vi "WILT Send Start Stop CMD.vi"(0 "Dryer Step 4 In":T5 {"Night Cycle Count" format="%04d"; "Day Cycle Count" format="%04d"}, 2 "Step 3 Input":T3, 3 "Final Start Presses":i32=2, 5 "Error In":errorcluster, 7 "Current Threshold":dbl, 8 "Station Number in":u32, 9 "Agilent Valve and Switch Locations":T2[](array[typedef])=[{"Channel"="301", "Station"="1", "Label"="Water Valve", "Agilent Station"="2", "Data"=0.0}, {"Channel"="302", "Station"="2", "Label"="Water Valve", "Agilent Station"="2", "Data"=0.0}, {"Channel"="303", "Station"="3", "Label"="Water Valve", "Agilent Station"="2", "Data"=0.0}, {"Channel"="304", "Station"="4", "Label"="Water Valve", "Agilent Station"="2", "Data"=0.0}, {"Channel"="305", "Station"="5", "Label"="Water Valve", "Agilent Station"="2", "Data"=0.0}, {"Channel"="306", "Station"="6", "Label"="Water Valve", "Agilent Station"="2", "Data"=0.0}, {"Channel"="307", "Station"="7", "Label"="Water Valve", "Agilent Station"="2", "Data"=0.0}, {"Channel"="308", "Station"="8", "Label"="Water Valve", "Agilent Station"="2", "Data"=0.0}, {"Channel"="309", "Station"="9", "Label"="Water Valve", "Agilent Station"="2", "Data"=0.0}, {"Channel"="310", "Station"="10", "Label"="Water Valve", "Agilent Station"="2", "Data"=0.0}, {"Channel"="311", "Station"="11", "Label"="Water Valve", "Agilent Station"="2", "Data"=0.0}, {"Channel"="312", "Station"="12", "Label"="Water Valve", "Agilent Station"="2", "Data"=0.0}, {"Channel"="313", "Station"="13", "Label"="Water Valve", "Agilent Station"="2", "Data"=0.0}, {"Channel"="314", "Station"="14", "Label"="Water Valve", "Agilent Station"="2", "Data"=0.0}, {"Channel"="315", "Station"="15", "Label"="Water Valve", "Agilent Station"="2", "Data"=0.0}, {"Channel"="316", "Station"="16", "Label"="Water Valve", "Agilent Station"="2", "Data"=0.0}, {"Channel"="317", "Station"="17", "Label"="Water Valve", "Agilent Station"="2", "Data"=0.0}, {"Channel"="318", "Station"="18", "Label"="Water Valve", "Agilent Station"="2", "Data"=0.0}, {"Channel"="319", "Station"="19", "Label"="Water Valve", "Agilent Station"="2", "Data"=0.0}, {"Channel"="320", "Station"="20", "Label"="Water Valve", "Agilent Station"="2", "Data"=0.0}, {"Channel"="101", "Station"="21", "Label"="Water Valve", "Agilent Station"="3", "Data"=0.0}, {"Channel"="102", "Station"="22", "Label"="Water Valve", "Agilent Station"="3", "Data"=0.0}, {"Channel"="103", "Station"="23", "Label"="Water Valve", "Agilent Station"="3", "Data"=0.0}, {"Channel"="104", "Station"="24", "Label"="Water Valve", "Agilent Station"="3", "Data"=0.0}, {"Channel"="105", "Station"="25", "Label"="Water Valve", "Agilent Station"="3", "Data"=0.0}, {"Channel"="106", "Station"="26", "Label"="Water Valve", "Agilent Station"="3", "Data"=0.0}, {"Channel"="107", "Station"="27", "Label"="Water Valve", "Agilent Station"="3", "Data"=0.0}, {"Channel"="108", "Station"="28", "Label"="Water Valve", "Agilent Station"="3", "Data"=0.0}, {"Channel"="109", "Station"="29", "Label"="Water Valve", "Agilent Station"="3", "Data"=0.0}, {"Channel"="110", "Station"="30", "Label"="Water Valve", "Agilent Station"="3", "Data"=0.0}, {"Channel"="111", "Station"="31", "Label"="Water Valve", "Agilent Station"="3", "Data"=0.0}, {"Channel"="112", "Station"="32", "Label"="Water Valve", "Agilent Station"="3", "Data"=0.0}, {"Channel"="101", "Station"="33", "Label"="Water Valve", "Agilent Station"="5", "Data"=0.0}, {"Channel"="102", "Station"="34", "Label"="Water Valve", "Agilent Station"="5", "Data"=0.0}, {"Channel"="103", "Station"="35", "Label"="Water Valve", "Agilent Station"="5", "Data"=0.0}, {"Channel"="104", "Station"="36", "Label"="Water Valve", "Agilent Station"="5", "Data"=0.0}, {"Channel"="105", "Station"="37", "Label"="Water Valve", "Agilent Station"="5", "Data"=0.0}, {"Channel"="106", "Station"="38", "Label"="Water Valve", "Agilent Station"="5", "Data"=0.0}, {"Channel"="107", "Station"="39", "Label"="Water Valve", "Agilent Station"="5", "Data"=0.0}, {"Channel"="108", "Station"="40", "Label"="Water Valve", "Agilent Station"="5", "Data"=0.0}, {"Channel"="109", "Station"="41", "Label"="Water Valve", "Agilent Station"="5", "Data"=0.0}, {"Channel"="110", "Station"="42", "Label"="Water Valve", "Agilent Station"="5", "Data"=0.0}, {"Channel"="111", "Station"="43", "Label"="Water Valve", "Agilent Station"="5", "Data"=0.0}, {"Channel"="112", "Station"="44", "Label"="Water Valve", "Agilent Station"="5", "Data"=0.0}, {"Channel"="113", "Station"="45", "Label"="Water Valve", "Agilent Station"="5", "Data"=0.0}, {"Channel"="114", "Station"="46", "Label"="Water Valve", "Agilent Station"="5", "Data"=0.0}, {"Channel"="115", "Station"="47", "Label"="Water Valve", "Agilent Station"="5", "Data"=0.0}, {"Channel"="116", "Station"="48", "Label"="Water Valve", "Agilent Station"="5", "Data"=0.0}, {"Channel"="117", "Station"="49", "Label"="Water Valve", "Agilent Station"="5", "Data"=0.0}, {"Channel"="118", "Station"="50", "Label"="Water Valve", "Agilent Station"="5", "Data"=0.0}, {"Channel"="119", "Station"="51", "Label"="Water Valve", "Agilent Station"="5", "Data"=0.0}, {"Channel"="120", "Station"="52", "Label"="Water Valve", "Agilent Station"="5", "Data"=0.0}, {"Channel"="201", "Station"="53", "Label"="Water Valve", "Agilent Station"="5", "Data"=0.0}, {"Channel"="202", "Station"="54", "Label"="Water Valve", "Agilent Station"="5", "Data"=0.0}, {"Channel"="203", "Station"="55", "Label"="Water Valve", "Agilent Station"="5", "Data"=0.0}, {"Channel"="204", "Station"="56", "Label"="Water Valve", "Agilent Station"="5", "Data"=0.0}, {"Channel"="301", "Station"="21", "Label"="Start Button", "Agilent Station"="5", "Data"=0.0}, {"Channel"="302", "Station"="22", "Label"="Start Button", "Agilent Station"="5", "Data"=0.0}, {"Channel"="303", "Station"="23", "Label"="Start Button", "Agilent Station"="5", "Data"=0.0}, {"Channel"="304", "Station"="24", "Label"="Start Button", "Agilent Station"="5", "Data"=0.0}, {"Channel"="305", "Station"="25", "Label"="Start Button", "Agilent Station"="5", "Data"=0.0}, {"Channel"="306", "Station"="26", "Label"="Start Button", "Agilent Station"="5", "Data"=0.0}, {"Channel"="307", "Station"="27", "Label"="Start Button", "Agilent Station"="5", "Data"=0.0}, {"Channel"="308", "Station"="28", "Label"="Start Button", "Agilent Station"="5", "Data"=0.0}, {"Channel"="309", "Station"="29", "Label"="Start Button", "Agilent Station"="5", "Data"=0.0}, {"Channel"="310", "Station"="30", "Label"="Start Button", "Agilent Station"="5", "Data"=0.0}, {"Channel"="311", "Station"="31", "Label"="Start Button", "Agilent Station"="5", "Data"=0.0}, {"Channel"="312", "Station"="32", "Label"="Start Button", "Agilent Station"="5", "Data"=0.0}, {"Channel"="101", "Station"="33", "Label"="Start Button", "Agilent Station"="7", "Data"=0.0}, {"Channel"="102", "Station"="34", "Label"="Start Button", "Agilent Station"="7", "Data"=0.0}, {"Channel"="103", "Station"="35", "Label"="Start Button", "Agilent Station"="7", "Data"=0.0}, {"Channel"="104", "Station"="36", "Label"="Start Button", "Agilent Station"="7", "Data"=0.0}, {"Channel"="105", "Station"="37", "Label"="Start Button", "Agilent Station"="7", "Data"=0.0}, {"Channel"="106", "Station"="38", "Label"="Start Button", "Agilent Station"="7", "Data"=0.0}, {"Channel"="107", "Station"="39", "Label"="Start Button", "Agilent Station"="7", "Data"=0.0}, {"Channel"="108", "Station"="40", "Label"="Start Button", "Agilent Station"="7", "Data"=0.0}, {"Channel"="109", "Station"="41", "Label"="Start Button", "Agilent Station"="7", "Data"=0.0}, {"Channel"="110", "Station"="42", "Label"="Start Button", "Agilent Station"="7", "Data"=0.0}, {"Channel"="111", "Station"="43", "Label"="Start Button", "Agilent Station"="7", "Data"=0.0}, {"Channel"="112", "Station"="44", "Label"="Start Button", "Agilent Station"="7", "Data"=0.0}, {"Channel"="113", "Station"="45", "Label"="Start Button", "Agilent Station"="7", "Data"=0.0}, {"Channel"="114", "Station"="46", "Label"="Start Button", "Agilent Station"="7", "Data"=0.0}, {"Channel"="115", "Station"="47", "Label"="Start Button", "Agilent Station"="7", "Data"=0.0}, {"Channel"="116", "Station"="48", "Label"="Start Button", "Agilent Station"="7", "Data"=0.0}, {"Channel"="117", "Station"="49", "Label"="Start Button", "Agilent Station"="7", "Data"=0.0}, {"Channel"="118", "Station"="50", "Label"="Start Button", "Agilent Station"="7", "Data"=0.0}, {"Channel"="119", "Station"="51", "Label"="Start Button", "Agilent Station"="7", "Data"=0.0}, {"Channel"="120", "Station"="52", "Label"="Start Button", "Agilent Station"="7", "Data"=0.0}, {"Channel"="201", "Station"="53", "Label"="Start Button", "Agilent Station"="7", "Data"=0.0}, {"Channel"="202", "Station"="54", "Label"="Start Button", "Agilent Station"="7", "Data"=0.0}, {"Channel"="203", "Station"="55", "Label"="Start Button", "Agilent Station"="7", "Data"=0.0}, {"Channel"="204", "Station"="56", "Label"="Start Button", "Agilent Station"="7", "Data"=0.0}], 13 "Semaphore":T1[](array[typedef])) -> (14 "Dryer Step 4 Output":T5 {"Night Cycle Count" format="%04d"; "Day Cycle Count" format="%04d"}, 16 "Step 3 Output":T3, 19 "Error Out":errorcluster)   [LabVIEW 2016]
uses:
  Type Definitions/WILT Station Test State Cluster.ctl
  Type Definitions/WILT Dryer Test State.ctl
  Type Definitions/WILT Dryer.ctl
  Type Definitions/WILT Dryer Details.ctl
  Type Definitions/WILT Agilent Channel Definition.ctl
  Type Definitions/WILT DAQ Data.ctl
  Globals/WILT Globals Main Program.vi
panel:
  # "Day"
  # "Night"
  # "Day"
  # "Night"
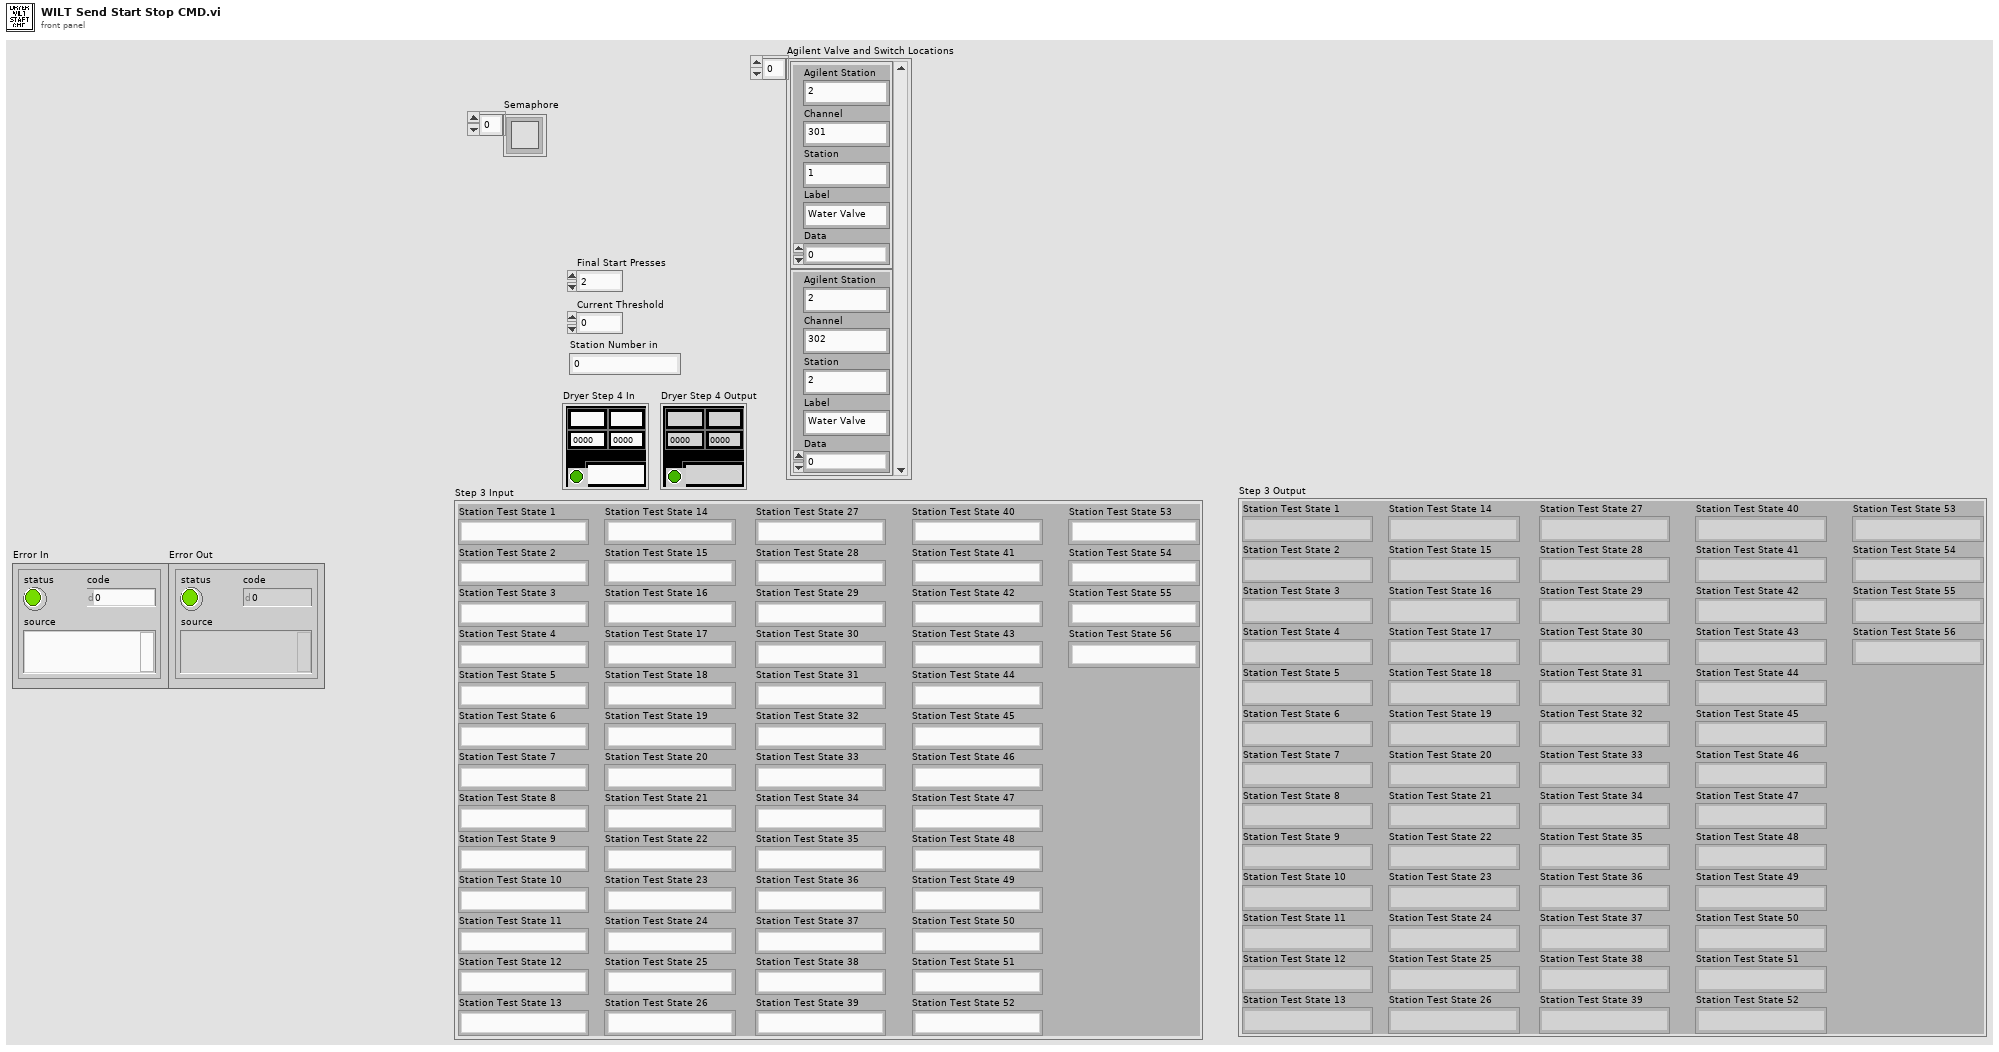
[diagram p1: front panel]
types:
  T1 = typedef "Semaphore RefNum" = refnum<k1>
  T2 = typedef "WILT Agilent Channel Definition.ctl" = cluster{"Channel":string, "Station":string, "Label":string, "Agilent Station":string, "Data":dbl}
  T3 = typedef "WILT Station Test State Cluster.ctl" = cluster{"Station Test State 1":T4, "Station Test State 2":T4, "Station Test State 3":T4, "Station Test State 4":T4, "Station Test State 5":T4, "Station Test State 6":T4, "Station Test State 7":T4, "Station Test State 8":T4, "Station Test State 9":T4, "Station Test State 10":T4, "Station Test State 11":T4, "Station Test State 12":T4, "Station Test State 13":T4, "Station Test State 14":T4, "Station Test State 15":T4, "Station Test State 16":T4, "Station Test State 17":T4, "Station Test State 18":T4, "Station Test State 19":T4, "Station Test State 20":T4, "Station Test State 21":T4, "Station Test State 22":T4, "Station Test State 23":T4, "Station Test State 24":T4, "Station Test State 25":T4, "Station Test State 26":T4, "Station Test State 27":T4, "Station Test State 28":T4, "Station Test State 29":T4, "Station Test State 30":T4, "Station Test State 31":T4, "Station Test State 32":T4, "Station Test State 33":T4, "Station Test State 34":T4, "Station Test State 35":T4, "Station Test State 36":T4, "Station Test State 37":T4, "Station Test State 38":T4, "Station Test State 39":T4, "Station Test State 40":T4, "Station Test State 41":T4, "Station Test State 42":T4, "Station Test State 43":T4, "Station Test State 44":T4, "Station Test State 45":T4, "Station Test State 46":T4, "Station Test State 47":T4, "Station Test State 48":T4, "Station Test State 49":T4, "Station Test State 50":T4, "Station Test State 51":T4, "Station Test State 52":T4, "Station Test State 53":T4, "Station Test State 54":T4, "Station Test State 55":T4, "Station Test State 56":T4}
  T4 = typedef "WILT Dryer Test State.ctl" = enum16{"No Serial Number", "Waiting for Dryer To Start", "Drying Clothes", "Water Injection 1 (On)", "Water Injection 1 Timer", "Water Injection 1 (Off)", "Pause Dryer", "Sending Start Stop CMD", "Pause Dryer 2", "Sending Start Stop CMD 2", "Drying Clothes 2", "Water Injection 2 (On)", "Water Injection 2 Timer", "Water Injection 2 (Off)", "Drying Clothes 3", "Cooling Down", "Sending Start Stop CMD 3", "Increment Cycle"}
  T5 = typedef "WILT Dryer.ctl" = cluster{"Lab ID":string, "Day Cycle Count":i32, "Station Label":string, "Dryer Details":T6, "Status Color":u32, "Invisible Button":bool, "Night Cycle Count":i32, "Station Index":i32, "Cycle Index":string, "Audit Alert":bool, "Agilent Channel Definition":T2, "DAQ Data":T7}
  T6 = typedef "WILT Dryer Details.ctl" = cluster{"Station":string, "Lab ID":string, "TR Number":string}
  T7 = typedef "WILT DAQ Data.ctl" = cluster{"L1 Current":dbl, "L2 Current":dbl, "Temperature  Deg F (TC)":dbl, "Volts":dbl, "Volts (208)":dbl, "SW (208)":dbl}
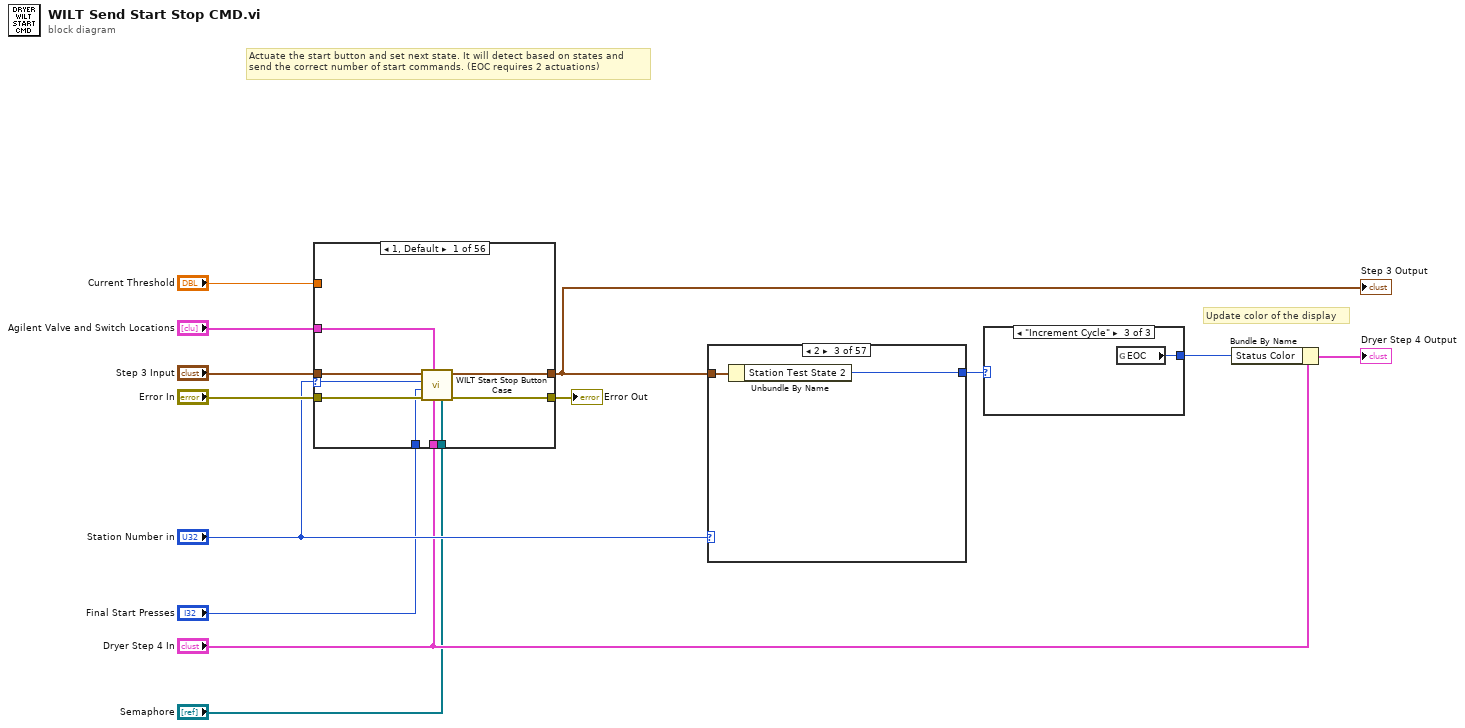
[diagram p0: block diagram]
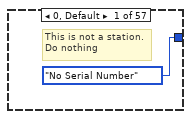
[diagram p2: hidden frame]
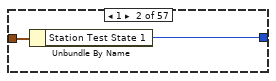
[diagram p3: hidden frame]
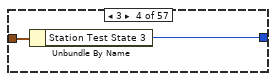
[diagram p4: hidden frame]
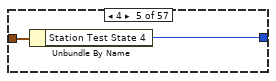
[diagram p5: hidden frame]
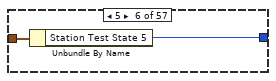
[diagram p6: hidden frame]
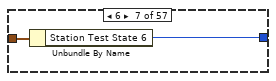
[diagram p7: hidden frame]
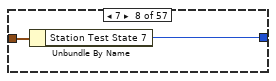
[diagram p8: hidden frame]
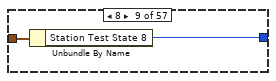
[diagram p9: hidden frame]
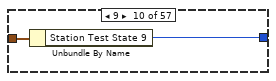
[diagram p10: hidden frame]
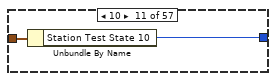
[diagram p11: hidden frame]
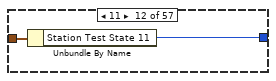
[diagram p12: hidden frame]
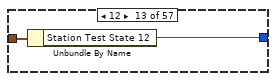
[diagram p13: hidden frame]
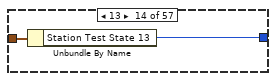
[diagram p14: hidden frame]
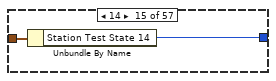
[diagram p15: hidden frame]
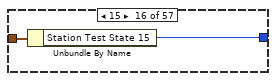
[diagram p16: hidden frame]
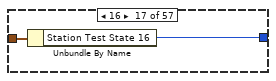
[diagram p17: hidden frame]
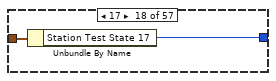
[diagram p18: hidden frame]
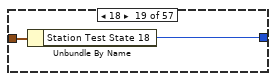
[diagram p19: hidden frame]
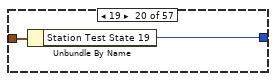
[diagram p20: hidden frame]
diagram:
  # "Update color of the display"
  # "Actuate the start button and set next state. It will detect based on states and \nsend the correct number of start commands. (EOC requires 2 actuations)"
  n1 = case shown="1, Default" "Station Number in" {
    selector: "Station Number in" -> [w20 w30 w38 w49 w58 w64 w72 w81 w90 w102 w109 w117 w128 w135 w144 w153 w162 w173 w180 w189 w198 w207 w216 w225 w238 w245 w254 w261 w273 w282 w290 w297 w309 w315 w324 w336 w342 w351 w360 w369 w380 w387 w399 w407 w416 w423 w432 w444 w450 w459 w468 w480 w486 w495 w504 w517]
    tunnel: "Step 3 Input" -> [w22 w31 w40 w48 w57 w65 w76 w85 w94 w103 w112 w121 w127 w139 w146 w157 w166 w175 w184 w193 w202 w211 w220 w229 w235 w247 w256 w265 w274 w283 w292 w301 w310 w319 w328 w337 w346 w355 w364 w371 w382 w391 w400 w409 w418 w427 w436 w445 w454 w463 w472 w481 w490 w499 w508 w516]
    tunnel: [w21 w27 w39 w47 w54 w63 w75 w84 w93 w99 w111 w120 w126 w136 w145 w156 w164 w172 w183 w192 w201 w210 w219 w228 w234 w244 w255 w264 w270 w279 w289 w300 w306 w318 w325 w333 w345 w354 w363 w370 w381 w390 w396 w408 w417 w426 w435 w441 w453 w462 w471 w477 w489 w498 w507 w515] -> w9
    tunnel: "Error In" -> [w19 w29 w37 w46 w56 w67 w73 w82 w91 w101 w110 w118 w130 w138 w148 w154 w165 w174 w181 w190 w199 w208 w217 w226 w237 w246 w253 w262 w272 w281 w291 w298 w308 w316 w327 w335 w343 w352 w361 w373 w379 w388 w398 w406 w415 w424 w433 w443 w451 w461 w469 w479 w487 w496 w505 w514]
    tunnel: [w18 w28 w36 w45 w55 w66 w74 w83 w92 w100 w108 w119 w129 w137 w147 w155 w163 w171 w182 w191 w200 w209 w218 w227 w236 w243 w252 w263 w271 w280 w288 w299 w307 w317 w326 w334 w344 w353 w362 w372 w378 w389 w397 w405 w414 w425 w434 w442 w452 w460 w470 w478 w488 w497 w506 w513] -> w10
    tunnel: "Agilent Valve and Switch Locations" -> [w17 w26 w35 w44 w53 w62 w71 w80 w89 w98 w107 w116 w125 w134 w143 w152 w161 w170 w179 w188 w197 w206 w215 w224 w233 w242 w251 w260 w269 w278 w287 w296 w305 w314 w323 w332 w341 w350 w359 w368 w377 w386 w395 w404 w413 w422 w431 w440 w449 w458 w467 w476 w485 w494 w503 w512]
    tunnel: "Current Threshold" -> [_ _ _ _ _ _ _ _ _ _ _ _ _ _ _ _ _ _ _ _ _ _ _ _ _ _ _ _ _ _ _ _ _ _ _ _ _ _ _ _ _ _ _ _ _ _ _ _ _ _ _ _ _ _ _ _]
    tunnel: "Dryer Step 4 In" -> [w16 w25 w34 w43 w52 w61 w70 w79 w88 w97 w106 w115 w124 w133 w142 w151 w160 w169 w178 w187 w196 w205 w214 w223 w232 w241 w250 w259 w268 w277 w286 w295 w304 w313 w322 w331 w340 w349 w358 w367 w376 w385 w394 w403 w412 w421 w430 w439 w448 w457 w466 w475 w484 w493 w502 w511]
    tunnel: "Semaphore" -> [w15 w24 w33 w42 w51 w60 w69 w78 w87 w96 w105 w114 w123 w132 w141 w150 w159 w168 w177 w186 w195 w204 w213 w222 w231 w240 w249 w258 w267 w276 w285 w294 w303 w312 w321 w330 w339 w348 w357 w366 w375 w384 w393 w402 w411 w420 w429 w438 w447 w456 w465 w474 w483 w492 w501 w510]
    tunnel: "Final Start Presses" -> [w14 w23 w32 w41 w50 w59 w68 w77 w86 w95 w104 w113 w122 w131 w140 w149 w158 w167 w176 w185 w194 w203 w212 w221 w230 w239 w248 w257 w266 w275 w284 w293 w302 w311 w320 w329 w338 w347 w356 w365 w374 w383 w392 w401 w410 w419 w428 w437 w446 w455 w464 w473 w482 w491 w500 w509]
    frame 1, Default {
      n2 = call "WILT Start Stop Button Case.vi"("Semaphore"=w15, "Dryer Step 4 In"=w16, "Agilent Valve and Switch Locations"=w17, "Error In"=w19, "Final Start Presses"=w14, "Station Number"=w20, "Step 3 Input in"=w22) -> ("Error Out"=w18:errorcluster, "Step 3 Input out"=w21:T3)  [unwired: 3 in]
    }
    frame 2 {
      n3 = call "WILT Start Stop Button Case.vi"("Semaphore"=w24, "Dryer Step 4 In"=w25, "Agilent Valve and Switch Locations"=w26, "Error In"=w29, "Final Start Presses"=w23, "Station Number"=w30, "Step 3 Input in"=w31) -> ("Error Out"=w28:errorcluster, "Step 3 Input out"=w27:T3)  [unwired: 3 in]
    }
    frame 3 {
      n4 = call "WILT Start Stop Button Case.vi"("Semaphore"=w33, "Dryer Step 4 In"=w34, "Agilent Valve and Switch Locations"=w35, "Error In"=w37, "Final Start Presses"=w32, "Station Number"=w38, "Step 3 Input in"=w40) -> ("Error Out"=w36:errorcluster, "Step 3 Input out"=w39:T3)  [unwired: 3 in]
    }
    frame 4 {
      n5 = call "WILT Start Stop Button Case.vi"("Semaphore"=w42, "Dryer Step 4 In"=w43, "Agilent Valve and Switch Locations"=w44, "Error In"=w46, "Final Start Presses"=w41, "Station Number"=w49, "Step 3 Input in"=w48) -> ("Error Out"=w45:errorcluster, "Step 3 Input out"=w47:T3)  [unwired: 3 in]
    }
    frame 5 {
      n6 = call "WILT Start Stop Button Case.vi"("Semaphore"=w51, "Dryer Step 4 In"=w52, "Agilent Valve and Switch Locations"=w53, "Error In"=w56, "Final Start Presses"=w50, "Station Number"=w58, "Step 3 Input in"=w57) -> ("Error Out"=w55:errorcluster, "Step 3 Input out"=w54:T3)  [unwired: 3 in]
    }
    frame 6 {
      n7 = call "WILT Start Stop Button Case.vi"("Semaphore"=w60, "Dryer Step 4 In"=w61, "Agilent Valve and Switch Locations"=w62, "Error In"=w67, "Final Start Presses"=w59, "Station Number"=w64, "Step 3 Input in"=w65) -> ("Error Out"=w66:errorcluster, "Step 3 Input out"=w63:T3)  [unwired: 3 in]
    }
    frame 7 {
      n8 = call "WILT Start Stop Button Case.vi"("Semaphore"=w69, "Dryer Step 4 In"=w70, "Agilent Valve and Switch Locations"=w71, "Error In"=w73, "Final Start Presses"=w68, "Station Number"=w72, "Step 3 Input in"=w76) -> ("Error Out"=w74:errorcluster, "Step 3 Input out"=w75:T3)  [unwired: 3 in]
    }
    frame 8 {
      n9 = call "WILT Start Stop Button Case.vi"("Semaphore"=w78, "Dryer Step 4 In"=w79, "Agilent Valve and Switch Locations"=w80, "Error In"=w82, "Final Start Presses"=w77, "Station Number"=w81, "Step 3 Input in"=w85) -> ("Error Out"=w83:errorcluster, "Step 3 Input out"=w84:T3)  [unwired: 3 in]
    }
    frame 9 {
      n10 = call "WILT Start Stop Button Case.vi"("Semaphore"=w87, "Dryer Step 4 In"=w88, "Agilent Valve and Switch Locations"=w89, "Error In"=w91, "Final Start Presses"=w86, "Station Number"=w90, "Step 3 Input in"=w94) -> ("Error Out"=w92:errorcluster, "Step 3 Input out"=w93:T3)  [unwired: 3 in]
    }
    frame 10 {
      n11 = call "WILT Start Stop Button Case.vi"("Semaphore"=w96, "Dryer Step 4 In"=w97, "Agilent Valve and Switch Locations"=w98, "Error In"=w101, "Final Start Presses"=w95, "Station Number"=w102, "Step 3 Input in"=w103) -> ("Error Out"=w100:errorcluster, "Step 3 Input out"=w99:T3)  [unwired: 3 in]
    }
    frame 11 {
      n12 = call "WILT Start Stop Button Case.vi"("Semaphore"=w105, "Dryer Step 4 In"=w106, "Agilent Valve and Switch Locations"=w107, "Error In"=w110, "Final Start Presses"=w104, "Station Number"=w109, "Step 3 Input in"=w112) -> ("Error Out"=w108:errorcluster, "Step 3 Input out"=w111:T3)  [unwired: 3 in]
    }
    frame 12 {
      n13 = call "WILT Start Stop Button Case.vi"("Semaphore"=w114, "Dryer Step 4 In"=w115, "Agilent Valve and Switch Locations"=w116, "Error In"=w118, "Final Start Presses"=w113, "Station Number"=w117, "Step 3 Input in"=w121) -> ("Error Out"=w119:errorcluster, "Step 3 Input out"=w120:T3)  [unwired: 3 in]
    }
    frame 13 {
      n14 = call "WILT Start Stop Button Case.vi"("Semaphore"=w123, "Dryer Step 4 In"=w124, "Agilent Valve and Switch Locations"=w125, "Error In"=w130, "Final Start Presses"=w122, "Station Number"=w128, "Step 3 Input in"=w127) -> ("Error Out"=w129:errorcluster, "Step 3 Input out"=w126:T3)  [unwired: 3 in]
    }
    frame 14 {
      n15 = call "WILT Start Stop Button Case.vi"("Semaphore"=w132, "Dryer Step 4 In"=w133, "Agilent Valve and Switch Locations"=w134, "Error In"=w138, "Final Start Presses"=w131, "Station Number"=w135, "Step 3 Input in"=w139) -> ("Error Out"=w137:errorcluster, "Step 3 Input out"=w136:T3)  [unwired: 3 in]
    }
    frame 15 {
      n16 = call "WILT Start Stop Button Case.vi"("Semaphore"=w141, "Dryer Step 4 In"=w142, "Agilent Valve and Switch Locations"=w143, "Error In"=w148, "Final Start Presses"=w140, "Station Number"=w144, "Step 3 Input in"=w146) -> ("Error Out"=w147:errorcluster, "Step 3 Input out"=w145:T3)  [unwired: 3 in]
    }
    frame 16 {
      n17 = call "WILT Start Stop Button Case.vi"("Semaphore"=w150, "Dryer Step 4 In"=w151, "Agilent Valve and Switch Locations"=w152, "Error In"=w154, "Final Start Presses"=w149, "Station Number"=w153, "Step 3 Input in"=w157) -> ("Error Out"=w155:errorcluster, "Step 3 Input out"=w156:T3)  [unwired: 3 in]
    }
    frame 17 {
      n18 = call "WILT Start Stop Button Case.vi"("Semaphore"=w159, "Dryer Step 4 In"=w160, "Agilent Valve and Switch Locations"=w161, "Error In"=w165, "Final Start Presses"=w158, "Station Number"=w162, "Step 3 Input in"=w166) -> ("Error Out"=w163:errorcluster, "Step 3 Input out"=w164:T3)  [unwired: 3 in]
    }
    frame 18 {
      n19 = call "WILT Start Stop Button Case.vi"("Semaphore"=w168, "Dryer Step 4 In"=w169, "Agilent Valve and Switch Locations"=w170, "Error In"=w174, "Final Start Presses"=w167, "Station Number"=w173, "Step 3 Input in"=w175) -> ("Error Out"=w171:errorcluster, "Step 3 Input out"=w172:T3)  [unwired: 3 in]
    }
    frame 19 {
      n20 = call "WILT Start Stop Button Case.vi"("Semaphore"=w177, "Dryer Step 4 In"=w178, "Agilent Valve and Switch Locations"=w179, "Error In"=w181, "Final Start Presses"=w176, "Station Number"=w180, "Step 3 Input in"=w184) -> ("Error Out"=w182:errorcluster, "Step 3 Input out"=w183:T3)  [unwired: 3 in]
    }
    frame 20 {
      n21 = call "WILT Start Stop Button Case.vi"("Semaphore"=w186, "Dryer Step 4 In"=w187, "Agilent Valve and Switch Locations"=w188, "Error In"=w190, "Final Start Presses"=w185, "Station Number"=w189, "Step 3 Input in"=w193) -> ("Error Out"=w191:errorcluster, "Step 3 Input out"=w192:T3)  [unwired: 3 in]
    }
    frame 21 {
      n22 = call "WILT Start Stop Button Case.vi"("Semaphore"=w195, "Dryer Step 4 In"=w196, "Agilent Valve and Switch Locations"=w197, "Error In"=w199, "Final Start Presses"=w194, "Station Number"=w198, "Step 3 Input in"=w202) -> ("Error Out"=w200:errorcluster, "Step 3 Input out"=w201:T3)  [unwired: 3 in]
    }
    frame 22 {
      n23 = call "WILT Start Stop Button Case.vi"("Semaphore"=w204, "Dryer Step 4 In"=w205, "Agilent Valve and Switch Locations"=w206, "Error In"=w208, "Final Start Presses"=w203, "Station Number"=w207, "Step 3 Input in"=w211) -> ("Error Out"=w209:errorcluster, "Step 3 Input out"=w210:T3)  [unwired: 3 in]
    }
    frame 23 {
      n24 = call "WILT Start Stop Button Case.vi"("Semaphore"=w213, "Dryer Step 4 In"=w214, "Agilent Valve and Switch Locations"=w215, "Error In"=w217, "Final Start Presses"=w212, "Station Number"=w216, "Step 3 Input in"=w220) -> ("Error Out"=w218:errorcluster, "Step 3 Input out"=w219:T3)  [unwired: 3 in]
    }
    frame 24 {
      n25 = call "WILT Start Stop Button Case.vi"("Semaphore"=w222, "Dryer Step 4 In"=w223, "Agilent Valve and Switch Locations"=w224, "Error In"=w226, "Final Start Presses"=w221, "Station Number"=w225, "Step 3 Input in"=w229) -> ("Error Out"=w227:errorcluster, "Step 3 Input out"=w228:T3)  [unwired: 3 in]
    }
    frame 25 {
      n26 = call "WILT Start Stop Button Case.vi"("Semaphore"=w231, "Dryer Step 4 In"=w232, "Agilent Valve and Switch Locations"=w233, "Error In"=w237, "Final Start Presses"=w230, "Station Number"=w238, "Step 3 Input in"=w235) -> ("Error Out"=w236:errorcluster, "Step 3 Input out"=w234:T3)  [unwired: 3 in]
    }
    frame 26 {
      n27 = call "WILT Start Stop Button Case.vi"("Semaphore"=w240, "Dryer Step 4 In"=w241, "Agilent Valve and Switch Locations"=w242, "Error In"=w246, "Final Start Presses"=w239, "Station Number"=w245, "Step 3 Input in"=w247) -> ("Error Out"=w243:errorcluster, "Step 3 Input out"=w244:T3)  [unwired: 3 in]
    }
    frame 27 {
      n28 = call "WILT Start Stop Button Case.vi"("Semaphore"=w249, "Dryer Step 4 In"=w250, "Agilent Valve and Switch Locations"=w251, "Error In"=w253, "Final Start Presses"=w248, "Station Number"=w254, "Step 3 Input in"=w256) -> ("Error Out"=w252:errorcluster, "Step 3 Input out"=w255:T3)  [unwired: 3 in]
    }
    frame 28 {
      n29 = call "WILT Start Stop Button Case.vi"("Semaphore"=w258, "Dryer Step 4 In"=w259, "Agilent Valve and Switch Locations"=w260, "Error In"=w262, "Final Start Presses"=w257, "Station Number"=w261, "Step 3 Input in"=w265) -> ("Error Out"=w263:errorcluster, "Step 3 Input out"=w264:T3)  [unwired: 3 in]
    }
    frame 29 {
      n30 = call "WILT Start Stop Button Case.vi"("Semaphore"=w267, "Dryer Step 4 In"=w268, "Agilent Valve and Switch Locations"=w269, "Error In"=w272, "Final Start Presses"=w266, "Station Number"=w273, "Step 3 Input in"=w274) -> ("Error Out"=w271:errorcluster, "Step 3 Input out"=w270:T3)  [unwired: 3 in]
    }
    frame 30 {
      n31 = call "WILT Start Stop Button Case.vi"("Semaphore"=w276, "Dryer Step 4 In"=w277, "Agilent Valve and Switch Locations"=w278, "Error In"=w281, "Final Start Presses"=w275, "Station Number"=w282, "Step 3 Input in"=w283) -> ("Error Out"=w280:errorcluster, "Step 3 Input out"=w279:T3)  [unwired: 3 in]
    }
    frame 31 {
      n32 = call "WILT Start Stop Button Case.vi"("Semaphore"=w285, "Dryer Step 4 In"=w286, "Agilent Valve and Switch Locations"=w287, "Error In"=w291, "Final Start Presses"=w284, "Station Number"=w290, "Step 3 Input in"=w292) -> ("Error Out"=w288:errorcluster, "Step 3 Input out"=w289:T3)  [unwired: 3 in]
    }
    frame 32 {
      n33 = call "WILT Start Stop Button Case.vi"("Semaphore"=w294, "Dryer Step 4 In"=w295, "Agilent Valve and Switch Locations"=w296, "Error In"=w298, "Final Start Presses"=w293, "Station Number"=w297, "Step 3 Input in"=w301) -> ("Error Out"=w299:errorcluster, "Step 3 Input out"=w300:T3)  [unwired: 3 in]
    }
    frame 33 {
      n34 = call "WILT Start Stop Button Case.vi"("Semaphore"=w303, "Dryer Step 4 In"=w304, "Agilent Valve and Switch Locations"=w305, "Error In"=w308, "Final Start Presses"=w302, "Station Number"=w309, "Step 3 Input in"=w310) -> ("Error Out"=w307:errorcluster, "Step 3 Input out"=w306:T3)  [unwired: 3 in]
    }
    frame 34 {
      n35 = call "WILT Start Stop Button Case.vi"("Semaphore"=w312, "Dryer Step 4 In"=w313, "Agilent Valve and Switch Locations"=w314, "Error In"=w316, "Final Start Presses"=w311, "Station Number"=w315, "Step 3 Input in"=w319) -> ("Error Out"=w317:errorcluster, "Step 3 Input out"=w318:T3)  [unwired: 3 in]
    }
    frame 35 {
      n36 = call "WILT Start Stop Button Case.vi"("Semaphore"=w321, "Dryer Step 4 In"=w322, "Agilent Valve and Switch Locations"=w323, "Error In"=w327, "Final Start Presses"=w320, "Station Number"=w324, "Step 3 Input in"=w328) -> ("Error Out"=w326:errorcluster, "Step 3 Input out"=w325:T3)  [unwired: 3 in]
    }
    frame 36 {
      n37 = call "WILT Start Stop Button Case.vi"("Semaphore"=w330, "Dryer Step 4 In"=w331, "Agilent Valve and Switch Locations"=w332, "Error In"=w335, "Final Start Presses"=w329, "Station Number"=w336, "Step 3 Input in"=w337) -> ("Error Out"=w334:errorcluster, "Step 3 Input out"=w333:T3)  [unwired: 3 in]
    }
    frame 37 {
      n38 = call "WILT Start Stop Button Case.vi"("Semaphore"=w339, "Dryer Step 4 In"=w340, "Agilent Valve and Switch Locations"=w341, "Error In"=w343, "Final Start Presses"=w338, "Station Number"=w342, "Step 3 Input in"=w346) -> ("Error Out"=w344:errorcluster, "Step 3 Input out"=w345:T3)  [unwired: 3 in]
    }
    frame 38 {
      n39 = call "WILT Start Stop Button Case.vi"("Semaphore"=w348, "Dryer Step 4 In"=w349, "Agilent Valve and Switch Locations"=w350, "Error In"=w352, "Final Start Presses"=w347, "Station Number"=w351, "Step 3 Input in"=w355) -> ("Error Out"=w353:errorcluster, "Step 3 Input out"=w354:T3)  [unwired: 3 in]
    }
    frame 39 {
      n40 = call "WILT Start Stop Button Case.vi"("Semaphore"=w357, "Dryer Step 4 In"=w358, "Agilent Valve and Switch Locations"=w359, "Error In"=w361, "Final Start Presses"=w356, "Station Number"=w360, "Step 3 Input in"=w364) -> ("Error Out"=w362:errorcluster, "Step 3 Input out"=w363:T3)  [unwired: 3 in]
    }
    frame 40 {
      n41 = call "WILT Start Stop Button Case.vi"("Semaphore"=w366, "Dryer Step 4 In"=w367, "Agilent Valve and Switch Locations"=w368, "Error In"=w373, "Final Start Presses"=w365, "Station Number"=w369, "Step 3 Input in"=w371) -> ("Error Out"=w372:errorcluster, "Step 3 Input out"=w370:T3)  [unwired: 3 in]
    }
    frame 41 {
      n42 = call "WILT Start Stop Button Case.vi"("Semaphore"=w375, "Dryer Step 4 In"=w376, "Agilent Valve and Switch Locations"=w377, "Error In"=w379, "Final Start Presses"=w374, "Station Number"=w380, "Step 3 Input in"=w382) -> ("Error Out"=w378:errorcluster, "Step 3 Input out"=w381:T3)  [unwired: 3 in]
    }
    frame 42 {
      n43 = call "WILT Start Stop Button Case.vi"("Semaphore"=w384, "Dryer Step 4 In"=w385, "Agilent Valve and Switch Locations"=w386, "Error In"=w388, "Final Start Presses"=w383, "Station Number"=w387, "Step 3 Input in"=w391) -> ("Error Out"=w389:errorcluster, "Step 3 Input out"=w390:T3)  [unwired: 3 in]
    }
    frame 43 {
      n44 = call "WILT Start Stop Button Case.vi"("Semaphore"=w393, "Dryer Step 4 In"=w394, "Agilent Valve and Switch Locations"=w395, "Error In"=w398, "Final Start Presses"=w392, "Station Number"=w399, "Step 3 Input in"=w400) -> ("Error Out"=w397:errorcluster, "Step 3 Input out"=w396:T3)  [unwired: 3 in]
    }
    frame 44 {
      n45 = call "WILT Start Stop Button Case.vi"("Semaphore"=w402, "Dryer Step 4 In"=w403, "Agilent Valve and Switch Locations"=w404, "Error In"=w406, "Final Start Presses"=w401, "Station Number"=w407, "Step 3 Input in"=w409) -> ("Error Out"=w405:errorcluster, "Step 3 Input out"=w408:T3)  [unwired: 3 in]
    }
    frame 45 {
      n46 = call "WILT Start Stop Button Case.vi"("Semaphore"=w411, "Dryer Step 4 In"=w412, "Agilent Valve and Switch Locations"=w413, "Error In"=w415, "Final Start Presses"=w410, "Station Number"=w416, "Step 3 Input in"=w418) -> ("Error Out"=w414:errorcluster, "Step 3 Input out"=w417:T3)  [unwired: 3 in]
    }
    frame 46 {
      n47 = call "WILT Start Stop Button Case.vi"("Semaphore"=w420, "Dryer Step 4 In"=w421, "Agilent Valve and Switch Locations"=w422, "Error In"=w424, "Final Start Presses"=w419, "Station Number"=w423, "Step 3 Input in"=w427) -> ("Error Out"=w425:errorcluster, "Step 3 Input out"=w426:T3)  [unwired: 3 in]
    }
    frame 47 {
      n48 = call "WILT Start Stop Button Case.vi"("Semaphore"=w429, "Dryer Step 4 In"=w430, "Agilent Valve and Switch Locations"=w431, "Error In"=w433, "Final Start Presses"=w428, "Station Number"=w432, "Step 3 Input in"=w436) -> ("Error Out"=w434:errorcluster, "Step 3 Input out"=w435:T3)  [unwired: 3 in]
    }
    frame 48 {
      n49 = call "WILT Start Stop Button Case.vi"("Semaphore"=w438, "Dryer Step 4 In"=w439, "Agilent Valve and Switch Locations"=w440, "Error In"=w443, "Final Start Presses"=w437, "Station Number"=w444, "Step 3 Input in"=w445) -> ("Error Out"=w442:errorcluster, "Step 3 Input out"=w441:T3)  [unwired: 3 in]
    }
    frame 49 {
      n50 = call "WILT Start Stop Button Case.vi"("Semaphore"=w447, "Dryer Step 4 In"=w448, "Agilent Valve and Switch Locations"=w449, "Error In"=w451, "Final Start Presses"=w446, "Station Number"=w450, "Step 3 Input in"=w454) -> ("Error Out"=w452:errorcluster, "Step 3 Input out"=w453:T3)  [unwired: 3 in]
    }
    frame 50 {
      n51 = call "WILT Start Stop Button Case.vi"("Semaphore"=w456, "Dryer Step 4 In"=w457, "Agilent Valve and Switch Locations"=w458, "Error In"=w461, "Final Start Presses"=w455, "Station Number"=w459, "Step 3 Input in"=w463) -> ("Error Out"=w460:errorcluster, "Step 3 Input out"=w462:T3)  [unwired: 3 in]
    }
    frame 51 {
      n52 = call "WILT Start Stop Button Case.vi"("Semaphore"=w465, "Dryer Step 4 In"=w466, "Agilent Valve and Switch Locations"=w467, "Error In"=w469, "Final Start Presses"=w464, "Station Number"=w468, "Step 3 Input in"=w472) -> ("Error Out"=w470:errorcluster, "Step 3 Input out"=w471:T3)  [unwired: 3 in]
    }
    frame 52 {
      n53 = call "WILT Start Stop Button Case.vi"("Semaphore"=w474, "Dryer Step 4 In"=w475, "Agilent Valve and Switch Locations"=w476, "Error In"=w479, "Final Start Presses"=w473, "Station Number"=w480, "Step 3 Input in"=w481) -> ("Error Out"=w478:errorcluster, "Step 3 Input out"=w477:T3)  [unwired: 3 in]
    }
    frame 53 {
      n54 = call "WILT Start Stop Button Case.vi"("Semaphore"=w483, "Dryer Step 4 In"=w484, "Agilent Valve and Switch Locations"=w485, "Error In"=w487, "Final Start Presses"=w482, "Station Number"=w486, "Step 3 Input in"=w490) -> ("Error Out"=w488:errorcluster, "Step 3 Input out"=w489:T3)  [unwired: 3 in]
    }
    frame 54 {
      n55 = call "WILT Start Stop Button Case.vi"("Semaphore"=w492, "Dryer Step 4 In"=w493, "Agilent Valve and Switch Locations"=w494, "Error In"=w496, "Final Start Presses"=w491, "Station Number"=w495, "Step 3 Input in"=w499) -> ("Error Out"=w497:errorcluster, "Step 3 Input out"=w498:T3)  [unwired: 3 in]
    }
    frame 55 {
      n56 = call "WILT Start Stop Button Case.vi"("Semaphore"=w501, "Dryer Step 4 In"=w502, "Agilent Valve and Switch Locations"=w503, "Error In"=w505, "Final Start Presses"=w500, "Station Number"=w504, "Step 3 Input in"=w508) -> ("Error Out"=w506:errorcluster, "Step 3 Input out"=w507:T3)  [unwired: 3 in]
    }
    frame 56 {
      n57 = call "WILT Start Stop Button Case.vi"("Semaphore"=w510, "Dryer Step 4 In"=w511, "Agilent Valve and Switch Locations"=w512, "Error In"=w514, "Final Start Presses"=w509, "Station Number"=w517, "Step 3 Input in"=w516) -> ("Error Out"=w513:errorcluster, "Step 3 Input out"=w515:T3)  [unwired: 3 in]
    }
  }
  "Error Out" <- w10
  "Step 3 Output" <- w9
  n58 = case shown="2" "Station Number in" {
    tunnel: w9 -> [_ w520 w522 w524 w526 w528 w530 w532 w534 w536 w538 w540 w542 w544 w546 w548 w550 w552 w554 w556 w558 w560 w562 w564 w566 w568 w570 w572 w574 w576 w578 w580 w582 w584 w586 w588 w590 w592 w594 w596 w598 w600 w602 w604 w606 w608 w610 w612 w614 w616 w618 w620 w622 w624 w626 w628 w630]
    tunnel: [WILT_Dryer_Test_State."No Serial Number" ("Station Test State 56") w519 w521 w523 w525 w527 w529 w531 w533 w535 w537 w539 w541 w543 w545 w547 w549 w551 w553 w555 w557 w559 w561 w563 w565 w567 w569 w571 w573 w575 w577 w579 w581 w583 w585 w587 w589 w591 w593 w595 w597 w599 w601 w603 w605 w607 w609 w611 w613 w615 w617 w619 w621 w623 w625 w627 w629] -> w7
    frame 0, Default {
      # "This is not a station.\nDo nothing"
    }
    frame 1 {
      n59 = Unbundle By Name(w520) -> ("Station Test State 1"=w519:T4)
    }
    frame 2 {
      n60 = Unbundle By Name(w522) -> ("Station Test State 2"=w521:T4)
    }
    frame 3 {
      n61 = Unbundle By Name(w524) -> ("Station Test State 3"=w523:T4)
    }
    frame 4 {
      n62 = Unbundle By Name(w526) -> ("Station Test State 4"=w525:T4)
    }
    frame 5 {
      n63 = Unbundle By Name(w528) -> ("Station Test State 5"=w527:T4)
    }
    frame 6 {
      n64 = Unbundle By Name(w530) -> ("Station Test State 6"=w529:T4)
    }
    frame 7 {
      n65 = Unbundle By Name(w532) -> ("Station Test State 7"=w531:T4)
    }
    frame 8 {
      n66 = Unbundle By Name(w534) -> ("Station Test State 8"=w533:T4)
    }
    frame 9 {
      n67 = Unbundle By Name(w536) -> ("Station Test State 9"=w535:T4)
    }
    frame 10 {
      n68 = Unbundle By Name(w538) -> ("Station Test State 10"=w537:T4)
    }
    frame 11 {
      n69 = Unbundle By Name(w540) -> ("Station Test State 11"=w539:T4)
    }
    frame 12 {
      n70 = Unbundle By Name(w542) -> ("Station Test State 12"=w541:T4)
    }
    frame 13 {
      n71 = Unbundle By Name(w544) -> ("Station Test State 13"=w543:T4)
    }
    frame 14 {
      n72 = Unbundle By Name(w546) -> ("Station Test State 14"=w545:T4)
    }
    frame 15 {
      n73 = Unbundle By Name(w548) -> ("Station Test State 15"=w547:T4)
    }
    frame 16 {
      n74 = Unbundle By Name(w550) -> ("Station Test State 16"=w549:T4)
    }
    frame 17 {
      n75 = Unbundle By Name(w552) -> ("Station Test State 17"=w551:T4)
    }
    frame 18 {
      n76 = Unbundle By Name(w554) -> ("Station Test State 18"=w553:T4)
    }
    frame 19 {
      n77 = Unbundle By Name(w556) -> ("Station Test State 19"=w555:T4)
    }
    frame 20 {
      n78 = Unbundle By Name(w558) -> ("Station Test State 20"=w557:T4)
    }
    frame 21 {
      n79 = Unbundle By Name(w560) -> ("Station Test State 21"=w559:T4)
    }
    frame 22 {
      n80 = Unbundle By Name(w562) -> ("Station Test State 22"=w561:T4)
    }
    frame 23 {
      n81 = Unbundle By Name(w564) -> ("Station Test State 23"=w563:T4)
    }
    frame 24 {
      n82 = Unbundle By Name(w566) -> ("Station Test State 24"=w565:T4)
    }
    frame 25 {
      n83 = Unbundle By Name(w568) -> ("Station Test State 25"=w567:T4)
    }
    frame 26 {
      n84 = Unbundle By Name(w570) -> ("Station Test State 26"=w569:T4)
    }
    frame 27 {
      n85 = Unbundle By Name(w572) -> ("Station Test State 27"=w571:T4)
    }
    frame 28 {
      n86 = Unbundle By Name(w574) -> ("Station Test State 28"=w573:T4)
    }
    frame 29 {
      n87 = Unbundle By Name(w576) -> ("Station Test State 29"=w575:T4)
    }
    frame 30 {
      n88 = Unbundle By Name(w578) -> ("Station Test State 30"=w577:T4)
    }
    frame 31 {
      n89 = Unbundle By Name(w580) -> ("Station Test State 31"=w579:T4)
    }
    frame 32 {
      n90 = Unbundle By Name(w582) -> ("Station Test State 32"=w581:T4)
    }
    frame 33 {
      n91 = Unbundle By Name(w584) -> ("Station Test State 33"=w583:T4)
    }
    frame 34 {
      n92 = Unbundle By Name(w586) -> ("Station Test State 34"=w585:T4)
    }
    frame 35 {
      n93 = Unbundle By Name(w588) -> ("Station Test State 35"=w587:T4)
    }
    frame 36 {
      n94 = Unbundle By Name(w590) -> ("Station Test State 36"=w589:T4)
    }
    frame 37 {
      n95 = Unbundle By Name(w592) -> ("Station Test State 37"=w591:T4)
    }
    frame 38 {
      n96 = Unbundle By Name(w594) -> ("Station Test State 38"=w593:T4)
    }
    frame 39 {
      n97 = Unbundle By Name(w596) -> ("Station Test State 39"=w595:T4)
    }
    frame 40 {
      n98 = Unbundle By Name(w598) -> ("Station Test State 40"=w597:T4)
    }
    frame 41 {
      n99 = Unbundle By Name(w600) -> ("Station Test State 41"=w599:T4)
    }
    frame 42 {
      n100 = Unbundle By Name(w602) -> ("Station Test State 42"=w601:T4)
    }
    frame 43 {
      n101 = Unbundle By Name(w604) -> ("Station Test State 43"=w603:T4)
    }
    frame 44 {
      n102 = Unbundle By Name(w606) -> ("Station Test State 44"=w605:T4)
    }
    frame 45 {
      n103 = Unbundle By Name(w608) -> ("Station Test State 45"=w607:T4)
    }
    frame 46 {
      n104 = Unbundle By Name(w610) -> ("Station Test State 46"=w609:T4)
    }
    frame 47 {
      n105 = Unbundle By Name(w612) -> ("Station Test State 47"=w611:T4)
    }
    frame 48 {
      n106 = Unbundle By Name(w614) -> ("Station Test State 48"=w613:T4)
    }
    frame 49 {
      n107 = Unbundle By Name(w616) -> ("Station Test State 49"=w615:T4)
    }
    frame 50 {
      n108 = Unbundle By Name(w618) -> ("Station Test State 50"=w617:T4)
    }
    frame 51 {
      n109 = Unbundle By Name(w620) -> ("Station Test State 51"=w619:T4)
    }
    frame 52 {
      n110 = Unbundle By Name(w622) -> ("Station Test State 52"=w621:T4)
    }
    frame 53 {
      n111 = Unbundle By Name(w624) -> ("Station Test State 53"=w623:T4)
    }
    frame 54 {
      n112 = Unbundle By Name(w626) -> ("Station Test State 54"=w625:T4)
    }
    frame 55 {
      n113 = Unbundle By Name(w628) -> ("Station Test State 55"=w627:T4)
    }
    frame 56 {
      n114 = Unbundle By Name(w630) -> ("Station Test State 56"=w629:T4)
    }
  }
  n115 = case shown="\"Increment Cycle\"" w7 {
    tunnel: [w631 w632 w633] -> w6
    frame "Pause Dryer 2", Default {
      n116 = global read "WILT Globals Main Program.vi" "Pause CMD 2"() -> (w631:u32)
    }
    frame "Drying Clothes 2" {
      n117 = global read "WILT Globals Main Program.vi" "Pause"() -> (w632:u32)
    }
    frame "Increment Cycle" {
      n118 = global read "WILT Globals Main Program.vi" "EOC"() -> (w633:u32)
    }
  }
  n119 = Bundle By Name(cluster="Dryer Step 4 In", "Status Color"=w6) -> (→"Dryer Step 4 Output":T5)
